vi "TracePoint_CameraDetected.vi"(8 "error in (no error)":errorcluster, 9 "new cameras":T1[](array[typedef]), 11 "Qbus":refnum<class "Qbus.lvclass">) -> (0 "error out":errorcluster)   [LabVIEW 2017, in "IrManageCameras.lvlib"]
uses:
  <vilib>/addons/InsightCM/Devices/Shared/Ir/IrManageCameras/IrManageCameras.lvlib
  <vilib>/addons/Qbus/Qbus.lvclass
  <vilib>/addons/InsightCM/Devices/Shared/Ir/IrManageCameras/controls/camera.ctl
  <vilib>/addons/TraceLogger/TraceLogger.lvlib
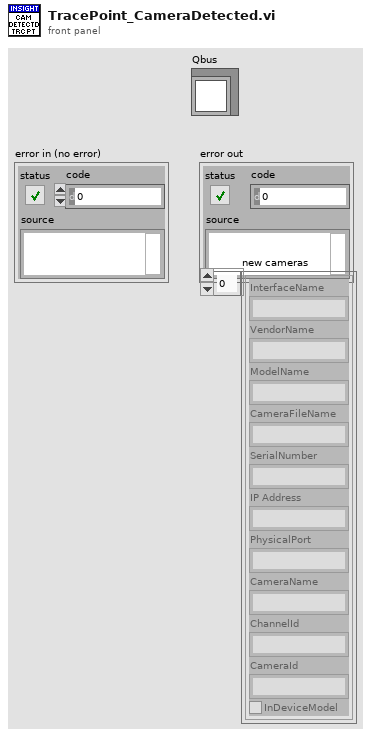
[diagram p1: front panel]
types:
  T1 = typedef "IrManageCameras.lvlib/camera.ctl" = cluster{"InterfaceName":string, "VendorName":string, "ModelName":string, "CameraFileName":string, "SerialNumber":string, "IP Address":string, "PhysicalPort":string, "CameraName":string, "ChannelId":string, "CameraId":string, "InDeviceModel":bool}
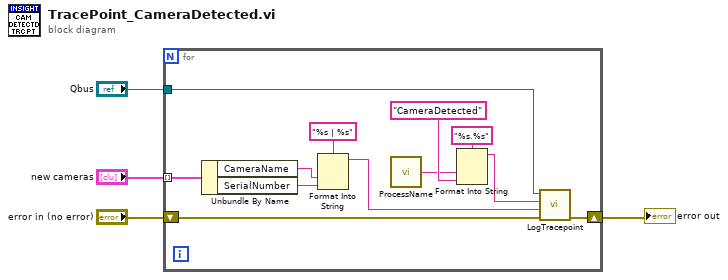
[diagram p0: block diagram]
diagram:
  n1 = for {
    tunnel: "new cameras" -> [w9] mode=indexing
    tunnel: "Qbus" -> [w8]
    shift-right: [w6] -> w1
    shift-left: "error in (no error)" -> [w7]
    n2 = Unbundle By Name(w9) -> ("CameraName"=w11:string, "SerialNumber"=w12:string)
    n3 = Format Into String(format string="%s | %s", w11, w12) -> (resulting string=w13:string)  [unwired: 2 in, 1 out]
    n4 = call <vilib>:"ProcessName.vi"() -> ("process name"=w5:string)  [unwired: 5 in]
    n5 = Format Into String(format string="%s.%s", w5, "CameraDetected" ("ProcessName")) -> (resulting string=w15:string)  [unwired: 2 in, 1 out]
    n6 = call <vilib>:"LogTracepoint.vi"("error in (no error)"=w7, "log string"=w13, "tracepoint"=w15, "qbus in"=w8) -> ("error out"=w6:errorcluster)  [unwired: 6 in, 1 out]
  }
  "error out" <- w1
